vi "ErrorQuery.vi"(8 "错误输入（无错误）":errorcluster, 11 "VISA引用句柄输入":refnum<visa-resource-name>) -> (0 "错误输出":errorcluster, 1 "全部错误消息":string, 2 "错误代码数组":i32[](array[numeric]), 3 "VISA引用句柄输出":refnum<visa-resource-name>)   [LabVIEW 2018]
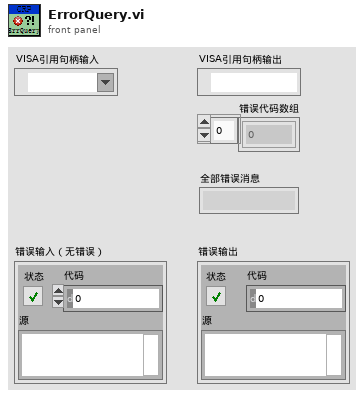
[diagram p1: front panel]
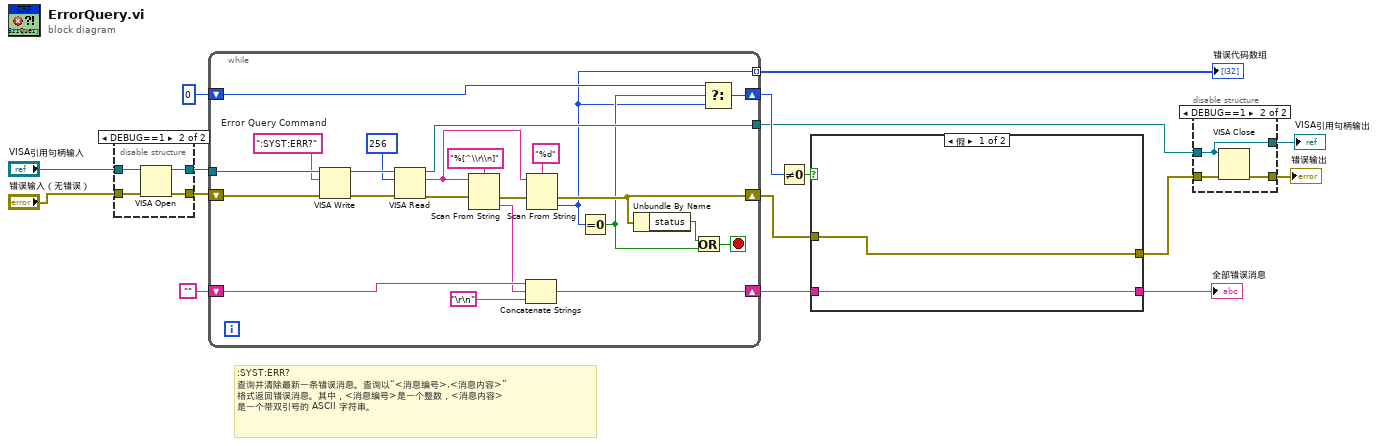
[diagram p0: block diagram]
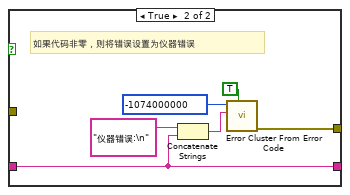
[diagram p4: hidden frame]
diagram:
  # ":SYST:ERR?\n查询并清除最新一条错误消息。查询以“<消息编号>,<消息内容>”\n格式返回错误消息。其中，<消息编号>是一个整数，<消息内容>\n是一个带双引号的 ASCII 字符串。"
  n1 = disable-structure shown="DEBUG==1" {
    disable-tunnel: [w18 w19] -> w8
    disable-tunnel: [w17 w20] -> w7
    disable-tunnel: "VISA引用句柄输入" -> [w18 w22]
    disable-tunnel: "错误输入（无错误）" -> [w17 w21]
    frame condition #0 {
    }
    frame condition #1 (active) {
      n2 = VISA Open(error in (no error)=w21, VISA resource name=w22) -> (VISA resource name=w19:refnum<visa-resource-name>, error out=w20:errorcluster)  [unwired: 3 in]
    }
  }
  n3 = while {
    tunnel: [w45] -> w4
    tunnel: w8 -> [w44]
    shift-right: [w23] -> w10
    shift-left: "" -> [w35]
    shift-right: [w32] -> w14
    shift-left: 0 -> [w33]
    shift-right: [w30] -> w16
    shift-left: w7 -> [w31]
    tunnel: [w24] -> w15 mode=indexing
    stop <- w38 stop-if-true
    w40 = ":SYST:ERR?"  # Error Query Command
    n4 = VISA Write(VISA resource name=w44, write buffer=w40, error in (no error)=w31) -> (VISA resource name out=w43:refnum<visa-resource-name>, error out=w41:errorcluster)  [unwired: 1 out]
    n5 = VISA Read(VISA resource name=w43, byte count=u32 256 ("Bytes"), error in (no error)=w41) -> (VISA resource name out=w45:refnum<visa-resource-name>, read buffer=w36:string, error out=w29:errorcluster)  [unwired: 1 out]
    n6 = Scan From String(format string="%[^\\r\\n]", input string=w36, error in=w29) -> (error out=w28:errorcluster, output 1=w34:string)  [unwired: 2 in, 2 out]
    n7 = Concatenate Strings(w35, w34, "\r\n") -> (w23:string)
    n8 = Scan From String(format string="%d", input string=w36, error in=w28) -> (error out=w30:errorcluster, output 1=w24:i32)  [unwired: 2 in, 2 out]
    n9 = Equal To 0?(x=w24) -> (x = 0?=w26:bool)
    n10 = Unbundle By Name(w30) -> ("status"=w27:bool)
    n11 = Or(x=w27, y=w26) -> (x .or. y?=w38:bool)
    n12 = Select(t=w33, s=w26, f=w24) -> (s? t:f=w32:i32)
  }
  "错误代码数组" <- w15
  n13 = Not Equal To 0?(x=w14) -> (x != 0?=w13:bool)
  n14 = case shown="假" w13 {
    tunnel: w10 -> [w46 w48]
    tunnel: [w47 w49] -> w3
    tunnel: w16 -> [w47 _]
    tunnel: [w46 w48] -> w9
    frame False {
    }
    frame True {
      # "如果代码非零，则将错误设置为仪器错误"
      n15 = Concatenate Strings("仪器错误:\n" ("Source"), w48) -> (w50:string)
      n16 = call <vilib>:"Error Cluster From Error Code.vi"("show call chain? (False)"=TRUE, "error message (\"\")"=w50, "error code (0)"=-1074000000 ("Code")) -> ("error out"=w49:errorcluster)  [unwired: 6 in]
    }
  }
  "全部错误消息" <- w9
  n17 = disable-structure shown="DEBUG==1" {
    disable-tunnel: w4 -> [w54 w56]
    disable-tunnel: w3 -> [w55 w58]
    disable-tunnel: [w55 w57] -> w2
    disable-tunnel: [w54 w56] -> w1
    frame condition #0 {
    }
    frame condition #1 (active) {
      n18 = VISA Close(VISA resource name=w56, error in (no error)=w58) -> (error out=w57:errorcluster)
    }
  }
  "错误输出" <- w2
  "VISA引用句柄输出" <- w1
